vi "run.vi"   [LabVIEW 2016, in "NURC2016.lvrbt"]
uses:
  NURC2016.lvrbt
  <vilib>/NXT/Block Support/NXT_InputPort.ctl
  <vilib>/NXT/Hardware/Plugins/Tetrix DC Motor/TetrixDCMotorAddress.ctl
  <vilib>/NXT/Hardware/Plugins/Tetrix 180 deg Servo/Tetrix180ServoAddress.ctl
  <vilib>/NXT/NXTIO Xnodes/NXTIONodeSubVIs/TETRIX IO Move Servos.vi
  <vilib>/NXT/Dual Mode Library/Waits/Wait_Num.vi
  <vilib>/NXT/NXTIO Xnodes/NXTIONodeSubVIs/TETRIX IO Move DC Motors.vi
  <vilib>/NXT/NXTIO Xnodes/NXTIONodeSubVIs/TETRIX IO Stop DC Motors.vi
  <vilib>/NXT/Dual Mode Library/Waits/Wait_EV3_Angle_Less.vi
  <vilib>/NXT/Dual Mode Library/Waits/Wait_EV3_Ultrasonic_Centimeter_Closer.vi
  <vilib>/NXT/Dual Mode Library/Waits/Wait_EV3_Angle_Greater.vi
  <vilib>/NXT/NXTIO Xnodes/AddressXNode/NXTIOAddress.xnode
  <vilib>/NXT/Subs/LVHSConnector.ctl
  <vilib>/NXT/NXTIO Xnodes/NXTIOXNode/NXTIO.xnode
  <vilib>/NXT/LegoClasses/BrickReference/BrickReference.lvclass
types:
  T1 = typedef "NXT_InputPort.ctl" = u32
  T2 = typedef "Tetrix180ServoAddress.ctl" = i32
  T3 = cluster{"Tetrix180Servo":T2, "Tetrix180Servo":T2, "Tetrix180Servo":T2}
  T4 = typedef "LVHSConnector.ctl" = refnum<class "BrickReference.lvclass">
  T5 = typedef "TetrixDCMotorAddress.ctl" = i32
  T6 = cluster{"Tetrix180Servo":T2, "Tetrix180Servo":T2}
diagram:
  w65 = T1 2 items=["Port 1", "Port 2", "Port 3", "Port 4"] ("Port (Port 1)")
  w107 = T1 2 items=["Port 1", "Port 2", "Port 3", "Port 4"] ("Port (Port 1)")
  w114 = T1 2 items=["Port 1", "Port 2", "Port 3", "Port 4"] ("Port (Port 1)")
  w160 = T1 2 items=["Port 1", "Port 2", "Port 3", "Port 4"] ("Port (Port 1)")
  w170 = T1 2 items=["Port 1", "Port 2", "Port 3", "Port 4"] ("Port (Port 1)")
  w180 = T1 2 items=["Port 1", "Port 2", "Port 3", "Port 4"] ("Port (Port 1)")
  w237 = T1 1 items=["Port 1", "Port 2", "Port 3", "Port 4"] ("Port (Port 1)")
  # "Extra  :\n\nMove foward to aim"
  # "Extra  :\n\nMove foward to aim"
  # "PART 12 :\n\nBack to base"
  # "PART 11 :\n\nTurn angle to back to base"
  # "PART 10 :\n\nMove backward to back to base"
  # "PART 9 :\n\nMove back to the rack"
  # "PART 8 :\n\nSecond  aim to the goal and ready to release"
  # "PART 7 :\n\nMove backward to detect the second ball and ready to grab the ball"
  # "PART 6 :\n\nBack to the rack to grab second ball"
  # "PART 5 :\n\nTurn to aim the goal and ready to release the ball"
  # "PART 4 :\n\nGrab the ball and ready to aim"
  # "PART 3 :\n\nMove straight to detect the ball"
  # "PART 2 :\n\nTurn to the left -70 Deg"
  # "PART 1 :\n\nMove straight out from the base"
  n1 = xnode "Motors"() -> ("Motor"=w218:T3)
  n2 = xnode "Move Servos"("Position 3"=u8 0, "Position 2"=u8 0, "Position 1"=u8 131, "Motors"=w218) -> ("NXT/EV3"=w188:T4)  [unwired: 1 in]
  n3 = xnode "Motors"() -> ("Motor"=w252:cluster{"TetrixDCMotor":T5, "TetrixDCMotor":T5})
  n4 = call-poly <vilib>:"PolyWait.vi"("Time (1 sec)"=sgl 1.0, "NXT/EV3"=w188) -> ("NXT/EV3"=w214:T4)  [unwired: 2 in]
  n5 = xnode "Move Motors"("Power/Speed 2"=i8 80, "Power/Speed 1"=i8 80, "Motors"=w252, "NXT/EV3"=w214) -> ("NXT/EV3"=w249:T4)
  n6 = xnode "Motors"() -> ("Motor"=w187:cluster{"TetrixDCMotor":T5, "TetrixDCMotor":T5})
  n7 = call-poly <vilib>:"PolyWait.vi"("Time (1 sec)"=sgl 1.0, "NXT/EV3"=w249) -> ("NXT/EV3"=w186:T4)  [unwired: 2 in]
  n8 = xnode "Stop Motors"("Motors"=w187, "NXT/EV3"=w186) -> ("NXT/EV3"=w185:T4)
  n9 = xnode "Motors"() -> ("Motor"=w246:cluster{"TetrixDCMotor":T5, "TetrixDCMotor":T5})
  n10 = call-poly <vilib>:"PolyWait.vi"("Time (1 sec)"=sgl 1.7, "NXT/EV3"=w185) -> ("NXT/EV3"=w243:T4)  [unwired: 2 in]
  n11 = xnode "Move Motors"("Power/Speed 2"=i8 0, "Power/Speed 1"=i8 30, "Motors"=w246, "NXT/EV3"=w243) -> ("NXT/EV3"=w182:T4)
  n12 = call <vilib>:"EV3_Gyro_Reset.vi"("NXT/EV3"=w182, "Port (Port 1)"=w180) -> ("NXT/EV3"=w181:T4)  [unwired: 2 in]
  n13 = call-poly <vilib>:"PolyWait.vi"("Degrees (180)"=sgl -70.0, "NXT/EV3"=w181, "Port (Port 1)"=w180) -> ("NXT/EV3"=w179:T4)  [unwired: 1 in]
  n14 = xnode "Motors"() -> ("Motor"=w184:cluster{"TetrixDCMotor":T5, "TetrixDCMotor":T5})
  n15 = xnode "Stop Motors"("Motors"=w184, "NXT/EV3"=w179) -> ("NXT/EV3"=w183:T4)
  n16 = xnode "Motors"() -> ("Motor"=w242:cluster{"TetrixDCMotor":T5, "TetrixDCMotor":T5})
  n17 = call-poly <vilib>:"PolyWait.vi"("Time (1 sec)"=sgl 2.0, "NXT/EV3"=w183) -> ("NXT/EV3"=w208:T4)  [unwired: 2 in]
  n18 = xnode "Move Motors"("Power/Speed 2"=i8 18, "Power/Speed 1"=i8 19, "Motors"=w242, "NXT/EV3"=w208) -> ("NXT/EV3"=w239:T4)
  n19 = call-poly <vilib>:"PolyWait.vi"("Centimeters (40)"=sgl 15.0, "NXT/EV3"=w239, "Port (Port 1)"=w237) -> ("NXT/EV3"=w236:T4)  [unwired: 1 in]
  n20 = xnode "Motors"() -> ("Motor"=w235:cluster{"TetrixDCMotor":T5, "TetrixDCMotor":T5})
  n21 = xnode "Stop Motors"("Motors"=w235, "NXT/EV3"=w236) -> ("NXT/EV3"=w234:T4)
  n22 = xnode "Motors"() -> ("Motor"=w231:T6)
  n23 = call-poly <vilib>:"PolyWait.vi"("Time (1 sec)"=sgl 1.0, "NXT/EV3"=w234) -> ("NXT/EV3"=w232:T4)  [unwired: 2 in]
  n24 = xnode "Move Servos"("Position 2"=u8 0, "Position 1"=u8 0, "Motors"=w231, "NXT/EV3"=w232) -> ("NXT/EV3"=w206:T4)
  n25 = xnode "Motors"() -> ("Motor"=w212:T2)
  n26 = call-poly <vilib>:"PolyWait.vi"("Time (1 sec)"=sgl 1.2, "NXT/EV3"=w206) -> ("NXT/EV3"=w205:T4)  [unwired: 2 in]
  n27 = xnode "Move Servos"("Position 1"=u8 49, "Motors"=w212, "NXT/EV3"=w205) -> ("NXT/EV3"=w210:T4)
  n28 = xnode "Motors"() -> ("Motor"=w227:T2)
  n29 = call-poly <vilib>:"PolyWait.vi"("Time (1 sec)"=sgl 1.8, "NXT/EV3"=w210) -> ("NXT/EV3"=w225:T4)  [unwired: 2 in]
  n30 = xnode "Move Servos"("Position 1"=u8 131, "Motors"=w227, "NXT/EV3"=w225) -> ("NXT/EV3"=w224:T4)
  n31 = xnode "Motors"() -> ("Motor"=w221:T2)
  n32 = call-poly <vilib>:"PolyWait.vi"("Time (1 sec)"=sgl 1.8, "NXT/EV3"=w224) -> ("NXT/EV3"=w22:T4)  [unwired: 2 in]
  n33 = xnode "Motors"() -> ("Motor"=w27:cluster{"TetrixDCMotor":T5, "TetrixDCMotor":T5})
  n34 = xnode "Motors"() -> ("Motor"=w177:T2)
  n35 = xnode "Move Motors"("Power/Speed 2"=i8 30, "Power/Speed 1"=i8 30, "Motors"=w27, "NXT/EV3"=w22) -> ("NXT/EV3"=w25:T4)
  n36 = xnode "Motors"() -> ("Motor"=w21:cluster{"TetrixDCMotor":T5, "TetrixDCMotor":T5})
  n37 = call-poly <vilib>:"PolyWait.vi"("Time (1 sec)"=sgl 0.5, "NXT/EV3"=w25) -> ("NXT/EV3"=w20:T4)  [unwired: 2 in]
  n38 = xnode "Motors"() -> ("Motor"=w189:cluster{"TetrixDCMotor":T5, "TetrixDCMotor":T5})
  n39 = xnode "Stop Motors"("Motors"=w21, "NXT/EV3"=w20) -> ("NXT/EV3"=w18:T4)
  n40 = call-poly <vilib>:"PolyWait.vi"("Time (1 sec)"=sgl 0.5, "NXT/EV3"=w18) -> ("NXT/EV3"=w17:T4)  [unwired: 2 in]
  n41 = xnode "Move Servos"("Position 1"=u8 160, "Motors"=w221, "NXT/EV3"=w17) -> ("NXT/EV3"=w219:T4)
  n42 = call-poly <vilib>:"PolyWait.vi"("Time (1 sec)"=sgl 1.4, "NXT/EV3"=w219) -> ("NXT/EV3"=w175:T4)  [unwired: 2 in]
  n43 = xnode "Move Servos"("Position 1"=u8 5, "Motors"=w177, "NXT/EV3"=w175) -> ("NXT/EV3"=w173:T4)
  n44 = call-poly <vilib>:"PolyWait.vi"("Time (1 sec)"=sgl 1.4, "NXT/EV3"=w173) -> ("NXT/EV3"=w16:T4)  [unwired: 2 in]
  n45 = xnode "Move Motors"("Power/Speed 2"=i8 0, "Power/Speed 1"=i8 30, "Motors"=w189, "NXT/EV3"=w16) -> ("NXT/EV3"=w169:T4)
  n46 = call <vilib>:"EV3_Gyro_Reset.vi"("NXT/EV3"=w169, "Port (Port 1)"=w170) -> ("NXT/EV3"=w172:T4)  [unwired: 2 in]
  n47 = xnode "Motors"() -> ("Motor"=w168:cluster{"TetrixDCMotor":T5, "TetrixDCMotor":T5})
  n48 = call-poly <vilib>:"PolyWait.vi"("Degrees (180)"=sgl -1.05, "NXT/EV3"=w172, "Port (Port 1)"=w170) -> ("NXT/EV3"=w167:T4)  [unwired: 1 in]
  n49 = xnode "Stop Motors"("Motors"=w168, "NXT/EV3"=w167) -> ("NXT/EV3"=w165:T4)
  n50 = xnode "Motors"() -> ("Motor"=w204:T6)
  n51 = call-poly <vilib>:"PolyWait.vi"("Time (1 sec)"=sgl 1.0, "NXT/EV3"=w165) -> ("NXT/EV3"=w164:T4)  [unwired: 2 in]
  n52 = xnode "Move Servos"("Position 2"=u8 5, "Position 1"=u8 131, "Motors"=w204, "NXT/EV3"=w164) -> ("NXT/EV3"=w201:T4)
  n53 = xnode "Motors"() -> ("Motor"=w198:T2)
  n54 = call-poly <vilib>:"PolyWait.vi"("Time (1 sec)"=sgl 1.0, "NXT/EV3"=w201) -> ("NXT/EV3"=w199:T4)  [unwired: 2 in]
  n55 = xnode "Move Servos"("Position 1"=u8 80, "Motors"=w198, "NXT/EV3"=w199) -> ("NXT/EV3"=w195:T4)
  n56 = xnode "Motors"() -> ("Motor"=w193:T2)
  n57 = call-poly <vilib>:"PolyWait.vi"("Time (1 sec)"=sgl 1.5, "NXT/EV3"=w195) -> ("NXT/EV3"=w192:T4)  [unwired: 2 in]
  n58 = xnode "Move Servos"("Position 1"=u8 0, "Motors"=w193, "NXT/EV3"=w192) -> ("NXT/EV3"=w153:T4)
  n59 = xnode "Motors"() -> ("Motor"=w157:cluster{"TetrixDCMotor":T5, "TetrixDCMotor":T5})
  n60 = call-poly <vilib>:"PolyWait.vi"("Time (1 sec)"=sgl 1.5, "NXT/EV3"=w153) -> ("NXT/EV3"=w152:T4)  [unwired: 2 in]
  n61 = xnode "Move Motors"("Power/Speed 2"=i8 0, "Power/Speed 1"=i8 -30, "Motors"=w157, "NXT/EV3"=w152) -> ("NXT/EV3"=w161:T4)
  n62 = call <vilib>:"EV3_Gyro_Reset.vi"("NXT/EV3"=w161, "Port (Port 1)"=w160) -> ("NXT/EV3"=w158:T4)  [unwired: 2 in]
  n63 = xnode "Motors"() -> ("Motor"=w162:cluster{"TetrixDCMotor":T5, "TetrixDCMotor":T5})
  n64 = call-poly <vilib>:"PolyWait.vi"("Degrees (180)"=sgl 1.05, "NXT/EV3"=w158, "Port (Port 1)"=w160) -> ("NXT/EV3"=w163:T4)  [unwired: 1 in]
  n65 = xnode "Stop Motors"("Motors"=w162, "NXT/EV3"=w163) -> ("NXT/EV3"=w145:T4)
  n66 = xnode "Motors"() -> ("Motor"=w146:cluster{"TetrixDCMotor":T5, "TetrixDCMotor":T5})
  n67 = call-poly <vilib>:"PolyWait.vi"("Time (1 sec)"=sgl 2.0, "NXT/EV3"=w145) -> ("NXT/EV3"=w151:T4)  [unwired: 2 in]
  n68 = xnode "Move Motors"("Power/Speed 2"=i8 -25, "Power/Speed 1"=i8 -25, "Motors"=w146, "NXT/EV3"=w151) -> ("NXT/EV3"=w39:T4)
  n69 = xnode "Motors"() -> ("Motor"=w33:cluster{"TetrixDCMotor":T5, "TetrixDCMotor":T5})
  n70 = call-poly <vilib>:"PolyWait.vi"("Time (1 sec)"=sgl 0.9, "NXT/EV3"=w39) -> ("NXT/EV3"=w34:T4)  [unwired: 2 in]
  n71 = xnode "Stop Motors"("Motors"=w33, "NXT/EV3"=w34) -> ("NXT/EV3"=w30:T4)
  n72 = xnode "Motors"() -> ("Motor"=w35:cluster{"TetrixDCMotor":T5, "TetrixDCMotor":T5})
  n73 = call-poly <vilib>:"PolyWait.vi"("Time (1 sec)"=sgl 1.0, "NXT/EV3"=w30) -> ("NXT/EV3"=w31:T4)  [unwired: 2 in]
  n74 = xnode "Move Motors"("Power/Speed 2"=i8 18, "Power/Speed 1"=i8 18, "Motors"=w35, "NXT/EV3"=w31) -> ("NXT/EV3"=w2:T4)
  n75 = call-poly <vilib>:"PolyWait.vi"("Time (1 sec)"=sgl 0.56 ("Centimeters (40)"), "NXT/EV3"=w2) -> ("NXT/EV3"=w1:T4)  [unwired: 2 in]
  n76 = xnode "Motors"() -> ("Motor"=w149:cluster{"TetrixDCMotor":T5, "TetrixDCMotor":T5})
  n77 = xnode "Stop Motors"("Motors"=w149, "NXT/EV3"=w1) -> ("NXT/EV3"=w120:T4)
  n78 = xnode "Motors"() -> ("Motor"=w123:T6)
  n79 = call-poly <vilib>:"PolyWait.vi"("Time (1 sec)"=sgl 1.0, "NXT/EV3"=w120) -> ("NXT/EV3"=w122:T4)  [unwired: 2 in]
  n80 = xnode "Move Servos"("Position 2"=u8 0, "Position 1"=u8 0, "Motors"=w123, "NXT/EV3"=w122) -> ("NXT/EV3"=w140:T4)
  n81 = xnode "Motors"() -> ("Motor"=w136:T2)
  n82 = call-poly <vilib>:"PolyWait.vi"("Time (1 sec)"=sgl 1.2, "NXT/EV3"=w140) -> ("NXT/EV3"=w141:T4)  [unwired: 2 in]
  n83 = xnode "Move Servos"("Position 1"=u8 49, "Motors"=w136, "NXT/EV3"=w141) -> ("NXT/EV3"=w138:T4)
  n84 = xnode "Motors"() -> ("Motor"=w127:T2)
  n85 = call-poly <vilib>:"PolyWait.vi"("Time (1 sec)"=sgl 1.8, "NXT/EV3"=w138) -> ("NXT/EV3"=w129:T4)  [unwired: 2 in]
  n86 = xnode "Move Servos"("Position 1"=u8 131, "Motors"=w127, "NXT/EV3"=w129) -> ("NXT/EV3"=w130:T4)
  n87 = xnode "Motors"() -> ("Motor"=w133:T2)
  n88 = xnode "Motors"() -> ("Motor"=w13:cluster{"TetrixDCMotor":T5, "TetrixDCMotor":T5})
  n89 = call-poly <vilib>:"PolyWait.vi"("Time (1 sec)"=sgl 1.8, "NXT/EV3"=w130) -> ("NXT/EV3"=w6:T4)  [unwired: 2 in]
  n90 = xnode "Move Motors"("Power/Speed 2"=i8 30, "Power/Speed 1"=i8 30, "Motors"=w13, "NXT/EV3"=w6) -> ("NXT/EV3"=w11:T4)
  n91 = xnode "Motors"() -> ("Motor"=w10:cluster{"TetrixDCMotor":T5, "TetrixDCMotor":T5})
  n92 = xnode "Motors"() -> ("Motor"=w142:T2)
  n93 = call-poly <vilib>:"PolyWait.vi"("Time (1 sec)"=sgl 0.3, "NXT/EV3"=w11) -> ("NXT/EV3"=w9:T4)  [unwired: 2 in]
  n94 = xnode "Stop Motors"("Motors"=w10, "NXT/EV3"=w9) -> ("NXT/EV3"=w7:T4)
  n95 = xnode "Motors"() -> ("Motor"=w117:cluster{"TetrixDCMotor":T5, "TetrixDCMotor":T5})
  n96 = call-poly <vilib>:"PolyWait.vi"("Time (1 sec)"=sgl 0.5, "NXT/EV3"=w7) -> ("NXT/EV3"=w5:T4)  [unwired: 2 in]
  n97 = xnode "Move Servos"("Position 1"=u8 160, "Motors"=w133, "NXT/EV3"=w5) -> ("NXT/EV3"=w135:T4)
  n98 = call-poly <vilib>:"PolyWait.vi"("Time (1 sec)"=sgl 1.4, "NXT/EV3"=w135) -> ("NXT/EV3"=w144:T4)  [unwired: 2 in]
  n99 = xnode "Move Servos"("Position 1"=u8 5, "Motors"=w142, "NXT/EV3"=w144) -> ("NXT/EV3"=w23:T4)
  n100 = call-poly <vilib>:"PolyWait.vi"("Time (1 sec)"=sgl 1.4, "NXT/EV3"=w23) -> ("NXT/EV3"=w4:T4)  [unwired: 2 in]
  n101 = xnode "Move Motors"("Power/Speed 2"=i8 0, "Power/Speed 1"=i8 30, "Motors"=w117, "NXT/EV3"=w4) -> ("NXT/EV3"=w113:T4)
  n102 = call <vilib>:"EV3_Gyro_Reset.vi"("NXT/EV3"=w113, "Port (Port 1)"=w114) -> ("NXT/EV3"=w116:T4)  [unwired: 2 in]
  n103 = xnode "Motors"() -> ("Motor"=w112:cluster{"TetrixDCMotor":T5, "TetrixDCMotor":T5})
  n104 = call-poly <vilib>:"PolyWait.vi"("Degrees (180)"=sgl -0.98, "NXT/EV3"=w116, "Port (Port 1)"=w114) -> ("NXT/EV3"=w111:T4)  [unwired: 1 in]
  n105 = xnode "Stop Motors"("Motors"=w112, "NXT/EV3"=w111) -> ("NXT/EV3"=w73:T4)
  n106 = xnode "Motors"() -> ("Motor"=w77:T6)
  n107 = call-poly <vilib>:"PolyWait.vi"("Time (1 sec)"=sgl 1.0, "NXT/EV3"=w73) -> ("NXT/EV3"=w91:T4)  [unwired: 2 in]
  n108 = xnode "Move Servos"("Position 2"=u8 5, "Position 1"=u8 131, "Motors"=w77, "NXT/EV3"=w91) -> ("NXT/EV3"=w80:T4)
  n109 = xnode "Motors"() -> ("Motor"=w83:T2)
  n110 = call-poly <vilib>:"PolyWait.vi"("Time (1 sec)"=sgl 6.0, "NXT/EV3"=w80) -> ("NXT/EV3"=w82:T4)  [unwired: 2 in]
  n111 = xnode "Move Servos"("Position 1"=u8 80, "Motors"=w83, "NXT/EV3"=w82) -> ("NXT/EV3"=w86:T4)
  n112 = xnode "Motors"() -> ("Motor"=w88:T2)
  n113 = call-poly <vilib>:"PolyWait.vi"("Time (1 sec)"=sgl 1.5, "NXT/EV3"=w86) -> ("NXT/EV3"=w89:T4)  [unwired: 2 in]
  n114 = xnode "Move Servos"("Position 1"=u8 0, "Motors"=w88, "NXT/EV3"=w89) -> ("NXT/EV3"=w75:T4)
  n115 = xnode "Motors"() -> ("Motor"=w104:cluster{"TetrixDCMotor":T5, "TetrixDCMotor":T5})
  n116 = call-poly <vilib>:"PolyWait.vi"("Time (1 sec)"=sgl 1.5, "NXT/EV3"=w75) -> ("NXT/EV3"=w74:T4)  [unwired: 2 in]
  n117 = xnode "Move Motors"("Power/Speed 2"=i8 0, "Power/Speed 1"=i8 -30, "Motors"=w104, "NXT/EV3"=w74) -> ("NXT/EV3"=w108:T4)
  n118 = call <vilib>:"EV3_Gyro_Reset.vi"("NXT/EV3"=w108, "Port (Port 1)"=w107) -> ("NXT/EV3"=w105:T4)  [unwired: 2 in]
  n119 = xnode "Motors"() -> ("Motor"=w109:cluster{"TetrixDCMotor":T5, "TetrixDCMotor":T5})
  n120 = call-poly <vilib>:"PolyWait.vi"("Degrees (180)"=sgl 0.98, "NXT/EV3"=w105, "Port (Port 1)"=w107) -> ("NXT/EV3"=w110:T4)  [unwired: 1 in]
  n121 = xnode "Stop Motors"("Motors"=w109, "NXT/EV3"=w110) -> ("NXT/EV3"=w100:T4)
  n122 = xnode "Motors"() -> ("Motor"=w97:cluster{"TetrixDCMotor":T5, "TetrixDCMotor":T5})
  n123 = call-poly <vilib>:"PolyWait.vi"("Time (1 sec)"=sgl 1.8, "NXT/EV3"=w100) -> ("NXT/EV3"=w96:T4)  [unwired: 2 in]
  n124 = xnode "Move Motors"("Power/Speed 2"=i8 -80, "Power/Speed 1"=i8 -80, "Motors"=w97, "NXT/EV3"=w96) -> ("NXT/EV3"=w94:T4)
  n125 = xnode "Motors"() -> ("Motor"=w93:cluster{"TetrixDCMotor":T5, "TetrixDCMotor":T5})
  n126 = call-poly <vilib>:"PolyWait.vi"("Time (1 sec)"=sgl 0.9, "NXT/EV3"=w94) -> ("NXT/EV3"=w92:T4)  [unwired: 2 in]
  n127 = xnode "Stop Motors"("Motors"=w93, "NXT/EV3"=w92) -> ("NXT/EV3"=w72:T4)
  n128 = xnode "Motors"() -> ("Motor"=w68:cluster{"TetrixDCMotor":T5, "TetrixDCMotor":T5})
  n129 = call-poly <vilib>:"PolyWait.vi"("Time (1 sec)"=sgl 1.0, "NXT/EV3"=w72) -> ("NXT/EV3"=w61:T4)  [unwired: 2 in]
  n130 = xnode "Move Motors"("Power/Speed 2"=i8 0, "Power/Speed 1"=i8 -30, "Motors"=w68, "NXT/EV3"=w61) -> ("NXT/EV3"=w64:T4)
  n131 = call <vilib>:"EV3_Gyro_Reset.vi"("NXT/EV3"=w64, "Port (Port 1)"=w65) -> ("NXT/EV3"=w67:T4)  [unwired: 2 in]
  n132 = xnode "Motors"() -> ("Motor"=w63:cluster{"TetrixDCMotor":T5, "TetrixDCMotor":T5})
  n133 = call-poly <vilib>:"PolyWait.vi"("Degrees (180)"=sgl 70.0, "NXT/EV3"=w67, "Port (Port 1)"=w65) -> ("NXT/EV3"=w62:T4)  [unwired: 1 in]
  n134 = xnode "Stop Motors"("Motors"=w63, "NXT/EV3"=w62) -> ("NXT/EV3"=w59:T4)
  n135 = xnode "Motors"() -> ("Motor"=w54:cluster{"TetrixDCMotor":T5, "TetrixDCMotor":T5})
  n136 = call-poly <vilib>:"PolyWait.vi"("Time (1 sec)"=sgl 1.0, "NXT/EV3"=w59) -> ("NXT/EV3"=w51:T4)  [unwired: 2 in]
  n137 = xnode "Move Motors"("Power/Speed 2"=i8 -80, "Power/Speed 1"=i8 -80, "Motors"=w54, "NXT/EV3"=w51) -> ("NXT/EV3"=w56:T4)
  n138 = xnode "Motors"() -> ("Motor"=w57:cluster{"TetrixDCMotor":T5, "TetrixDCMotor":T5})
  n139 = call-poly <vilib>:"PolyWait.vi"("Time (1 sec)"=sgl 0.9, "NXT/EV3"=w56) -> ("NXT/EV3"=w58:T4)  [unwired: 2 in]
  n140 = xnode "Stop Motors"("Motors"=w57, "NXT/EV3"=w58) -> ("NXT/EV3"=w50:T4)
  n141 = xnode "Motors"() -> ("Motor"=w47:T6)
  n142 = call-poly <vilib>:"PolyWait.vi"("Time (1 sec)"=sgl 1.0, "NXT/EV3"=w50) -> ("NXT/EV3"=w48:T4)  [unwired: 2 in]
  n143 = xnode "Move Servos"("Position 2"=u8 0, "Position 1"=u8 5, "Motors"=w47, "NXT/EV3"=w48) -> ("NXT/EV3"=w43:T4)
  n144 = xnode "Motors"() -> ("Motor"=w41:T2)
  n145 = call-poly <vilib>:"PolyWait.vi"("Time (1 sec)"=sgl 0.5, "NXT/EV3"=w43) -> ("NXT/EV3"=w42:T4)  [unwired: 2 in]
  n146 = xnode "Move Servos"("Position 1"=u8 0, "Motors"=w41, "NXT/EV3"=w42) -> ()  [unwired: 1 out]
